vi "send record.vi"(8 "error in":errorcluster, 9 "data":string, 10 "header":T1, 11 "connection":refnum<k5>) -> (0 "error out":errorcluster)   [LabVIEW 2013]
uses:
  record header.ctl
  record types.ctl
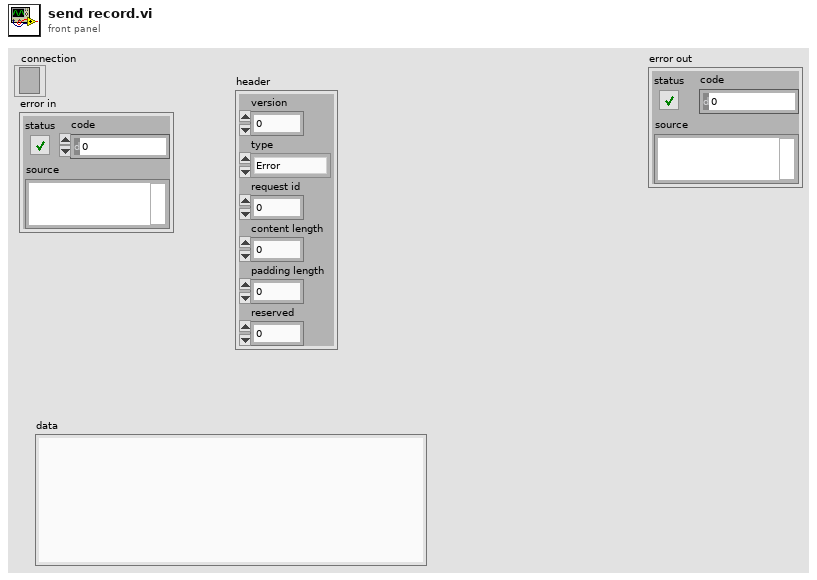
[diagram p1: front panel]
types:
  T1 = typedef "record header.ctl" = cluster{"version":u8, "type":T2, "request id":u16, "content length":u16, "padding length":u8, "reserved":u8}
  T2 = typedef "record types.ctl" = enum8{"Error", "Begin Request", "Abort Request", "End Request", "Parameters", "Standard Input", "Standard Output", "Standard Error", "Data", "Get Values", "Get Values Result", "Unknown Type"}
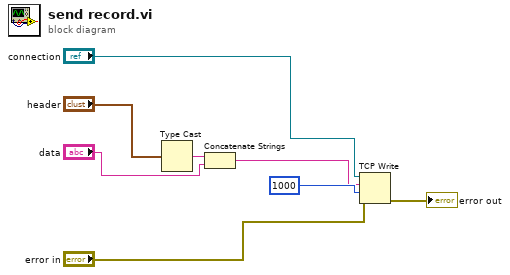
[diagram p0: block diagram]
diagram:
  n1 = Type Cast(x="header") -> (*(type *) &x=w2:string)  [unwired: 1 in]
  n2 = Concatenate Strings(w2, "data") -> (w1:string)
  n3 = TCP Write(connection ID="connection", data in=w1, error in (no error)="error in", 9:1000 ("timeout ms (25000)")) -> (error out=→"error out":errorcluster)  [unwired: 2 out]
